vi "Initialize.vi"(6 "optional":variant, 8 "error in (no error)":errorcluster, 11 "Graph in":refnum<class "Graph.lvclass">) -> (0 "error out":errorcluster, 3 "Graph out":refnum<class "Graph.lvclass">)   [LabVIEW 2009, in "Graph.lvclass"]
uses:
  Graph.lvclass
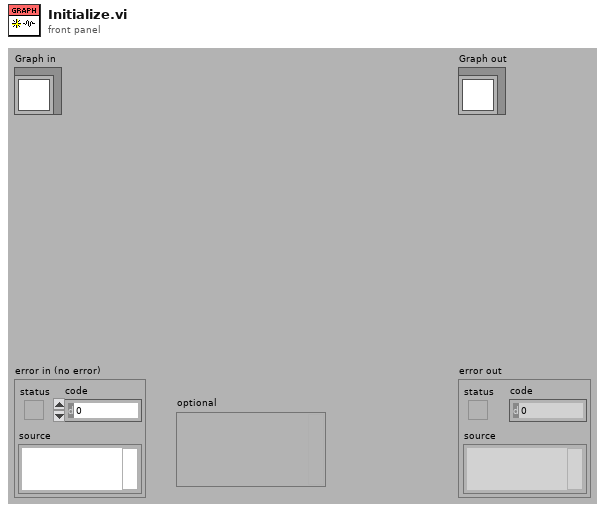
[diagram p1: front panel]
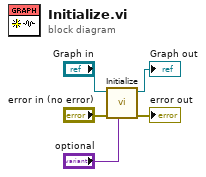
[diagram p0: block diagram]
diagram:
  n1 = call-parent "Initialize.vi"("optional"="optional", "error in (no error)"="error in (no error)", "Structure in"="Graph in") -> ("error out"=→"error out":errorcluster, "Structure out"=→"Graph out":refnum<class "Graph.lvclass">)  [unwired: 7 in]
